vi "S2C_Access_Open.vi"(8 "Error In":errorcluster, 11 "DSN_Path":path) -> (0 "Error Out":errorcluster, 3 "DB_Ref":T1)   [LabVIEW 2015]
uses:
  <vilib>/addons/database/Connection.llb/Conn ObjectReference.ctl
  <vilib>/addons/database/Connection.llb/DB Tools Open Connec (Path).vi
  S2C_Access_Globals.vi
  <vilib>/addons/database/NI_Database_API.lvlib
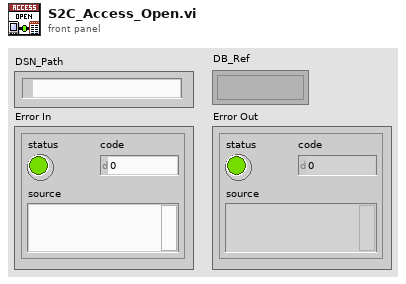
[diagram p1: front panel]
types:
  T1 = typedef "NI_Database_API.lvlib/Conn ObjectReference.ctl" = refnum<k1>
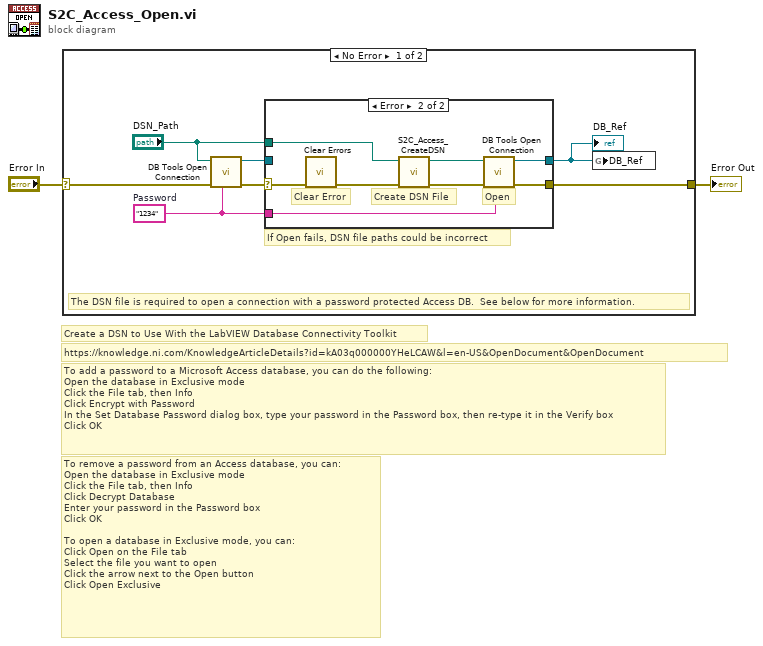
[diagram p0: block diagram]
diagram:
  # "To add a password to a Microsoft Access database, you can do the following:\nOpen the database in Exclusive mode\nClick the File tab, then Info\nClick Encrypt with Password\nIn the Set Database Password dialog box, type your password in the Password box, then re-type it in the Verify box\nClick OK"
  # "To remove a password from an Access database, you can:\nOpen the database in Exclusive mode\nClick the File tab, then Info\nClick Decrypt Database\nEnter your password in the Password box\nClick OK\n \nTo open a database in Exclusive mode, you can:\nClick Open on the File tab\nSelect the file you want to open\nClick the arrow next to the Open button\nClick Open Exclusive"
  # "Create a DSN to Use With the LabVIEW Database Connectivity Toolkit"
  # "https://knowledge.ni.com/KnowledgeArticleDetails?id=kA03q000000YHeLCAW&l=en-US&OpenDocument&OpenDocument"
  n1 = case shown="No Error" "Error In" {
    selector: "Error In" -> [w9 w20]
    tunnel: [w6 w20] -> w1
    frame No Error {
      w4 = "1234"  # Password
      # "If Open fails, DSN file paths could be incorrect"
      # "The DSN file is required to open a connection with a password protected Access DB.  See below for more information."
      n2 = call-poly <vilib>:"DB Tools Open Connection.vi"("password"=w4, "error in (no error)"=w9, "connection information"="DSN_Path") -> ("error out"=w8:errorcluster, "connection reference"=w7:T1)  [unwired: 5 in]
      n3 = case shown="Error" w8 {
        selector: w8 -> [w11 w19]
        tunnel: w7 -> [w10 _]
        tunnel: "DSN_Path" -> [_ w17]
        tunnel: [w10 w14] -> w5
        tunnel: [w11 w13] -> w6
        tunnel: w4 -> [_ w12]
        frame No Error {
        }
        frame Error {
          # "Open"
          # "Create DSN File"
          # "Clear Error"
          n4 = call <vilib>:"Clear Errors.vi"("error in (no error)"=w19) -> ("error out"=w18:errorcluster)  [unwired: 5 in, 1 out]
          n5 = call "S2C_Access_CreateDSN.vi"("Error In"=w18, "Path In"=w17) -> ("Error Out"=w16:errorcluster, "Path Out"=w15:path)  [unwired: 8 in]
          n6 = call-poly <vilib>:"DB Tools Open Connection.vi"("password"=w12, "error in (no error)"=w16, "connection information"=w15) -> ("error out"=w13:errorcluster, "connection reference"=w14:T1)  [unwired: 5 in]
        }
      }
      "DB_Ref" <- w5
      n7 = global write "S2C_Access_Globals.vi" "DB_Ref"(w5) -> ()
    }
    frame Error {
    }
  }
  "Error Out" <- w1
